vi "EdgeDetection-Simple.vi"() -> ()   [LabVIEW 2014]
doc: "This example shows how to use the Edge Tool in NI Vision. The Edge Tool finds edges (or sharp transitions in the pixels values) along a given line or ROI profile. The Edge Tool is a precursor function to many of the gauging and inspection tasks. For example, the location of the edges found along a line profile across an object can interpreted as the boundaries of the object whose dimensions have to be measured for a gauging application or the presence of a crack in the surface of an object for an inspection application."
uses:
  <vilib>/vision/NI_Vision_Development_Module.lvlib
panel:
  in  "Process":u16(ring)=2 items=["Get First Edge", "Get First + Last Edge", "Get All Edges"]
  in  "Threshold Parameters":T1={"Level Type"=enum."Absolute Value", "Threshold Level"=200, "Hysteresis"=10}
  out "Number of Edges Detected":i32
  out "Image":T2(plugin-control)
  out "Line Profile":cluster{"x0":sgl, "dx":sgl, "Pixels Line":sgl[]}(graph)
  in  "Stop":bool
  # "Instruction:\nThreshold Level can be either absolute or relative. \nAbsolute threshold is based on the pixel values. \nRelative threshold is expressed as a percentage of the pixel-value range found along the path defined by the pixel coordinates."
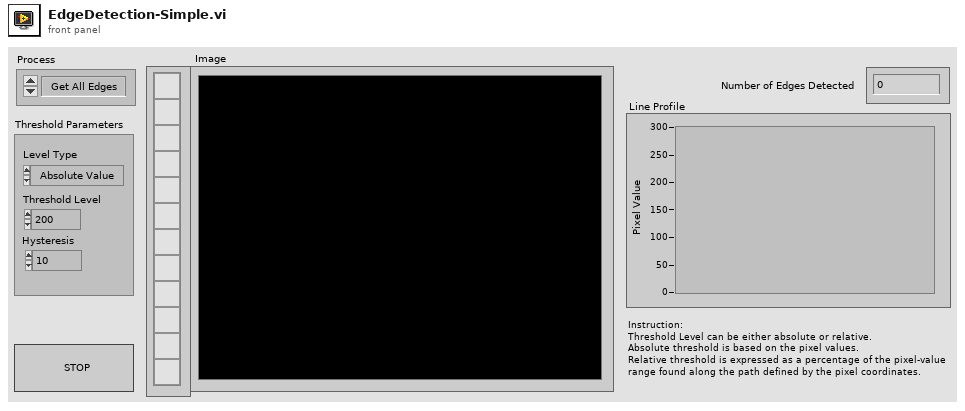
[diagram p1: front panel]
types:
  T1 = cluster{"Level Type":enum32{"Absolute Value", "Relative value"}, "Threshold Level":i32, "Hysteresis":i32}
  T2 = typedef "IMAQ Image.ctl" = refnum<image>
  T3 = typedef "IMAQ Line" = cluster{"Start X":i32, "Start Y":i32, "End X":i32, "End Y":i32}
  T4 = typedef "ROI Descriptor" = cluster{"Global Rectangle":i32[], "Contours":cluster{"ID":enum32{"External", "Internal"}, "Type":u32, "Coordinates":i32[]}[]}
  T5 = cluster{"Global Rectangle":i32[], "Contours":cluster{"Contour Type":u32, "ROI Type":u32, "Points":i32[]}[]}
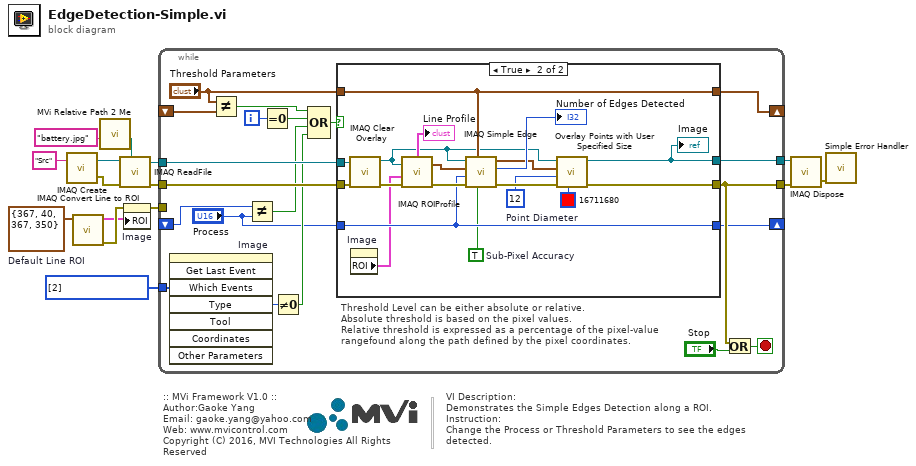
[diagram p0: block diagram]
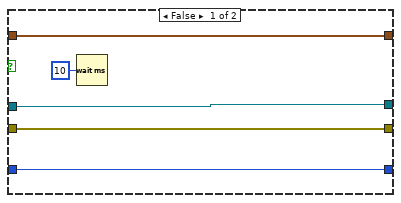
[diagram p2: hidden frame]
diagram:
  w4 = i32[] [2] items=["No Event"=0, "Click Event"=1, "Draw Event"=2, "Size Event"=4, "Scroll Event"=5, "Double Click Event"=8] ("Which Events")
  w7 = T3 {"Start X"=367, "Start Y"=40, "End X"=367, "End Y"=350}  # Default Line ROI
  # "VI Description:\nDemonstrates the Simple Edges Detection along a ROI.\nInstruction:\nChange the Process or Threshold Parameters to see the edges detected."
  # ":: MVi Framework V1.0 ::\nAuthor:Gaoke Yang\nEmail: gaoke.yang@yahoo.com\nWeb: www.mvicontrol.com\nCopyright (C) 2016, MVI Technologies All Rights Reserved"
  n1 = call "IMAQ Create"("Image Name"="Src") -> ("New Image"=w14:T2, "error out"=w13:errorcluster)  [unwired: 4 in]
  n2 = call "IMAQ Convert Line to ROI"("Line"=w7) -> ("error out"=w3:errorcluster, "ROI Descriptor"=w2:T4)  [unwired: 8 in]
  n3 = call "MVi Relative Path 2 Me.vi"("Relative Path"="battery.jpg" ("name or relative path")) -> ("Appended Dir"=w5:path)  [unwired: 5 in, 1 out]
  n4 = call "IMAQ ReadFile"("File Path"=w5, "error in (no error)"=w13, "Image"=w14) -> ("error out"=w8:errorcluster, "Image Out"=w9:T2)  [unwired: 4 in, 3 out]
  n5 = property on="Image" class="ImageControl"(error in=w3, "ROI"=w2) -> (error out=w1:errorcluster)  [unwired: 1 in, 1 out]
  n6 = while {
    tunnel: w9 -> [w34]
    tunnel: w8 -> [w35]
    tunnel: [w30] -> w12
    tunnel: [w31] -> w11
    shift-right: [w28] -> _
    shift-left: _ -> [w26]
    shift-right: [w25] -> _
    shift-left: _ -> [w19]
    tunnel: w4 -> [w24]
    tunnel: w1 -> [_]
    i -> [w29]
    stop <- w32 stop-if-true
    # "Threshold Level can be either absolute or relative. \nAbsolute threshold is based on the pixel values. \nRelative threshold is expressed as a percentage of the pixel-value\nrangefound along the path defined by the pixel coordinates."
    n7 = invoke on="Image" class="ImageControl" method="Get Last Event"("Which Events"=w24) -> ("Type"=w23:i32)  [unwired: 7 in, 7 out]
    n8 = Not Equal?(x="Threshold Parameters", y=w26) -> (x != y?=w20:bool)
    n9 = Not Equal?(x=w19, y="Process") -> (x != y?=w16:bool)
    n10 = Equal To 0?(x=w29) -> (x = 0?=w17:bool)
    n11 = Not Equal To 0?(x=w23) -> (x != 0?=w21:bool)
    n12 = Compound Arithmetic op=OR(w20, w17, w16, w21) -> (w22:bool)
    n13 = case shown="True" w22 {
      tunnel: w35 -> [w39 w47]
      tunnel: w34 -> [w40 w48]
      tunnel: [w40 w49] -> w31
      tunnel: [w39 w51] -> w30
      tunnel: "Threshold Parameters" -> [w37 w56]
      tunnel: [w37 w56] -> w28
      tunnel: "Process" -> [w36 w43]
      tunnel: [w36 w43] -> w25
      frame False {
        n14 = Wait (ms)(milliseconds to wait=u32 10) -> ()  [unwired: 1 out]
      }
      frame True {
        w42 = TRUE  # Sub-Pixel Accuracy
        w44 = u32 12  # Point Diameter
        n15 = call "IMAQ Clear Overlay"("error in (no error)"=w47, "Image"=w48) -> ("error out"=w46:errorcluster, "Image Out"=w45:T2)  [unwired: 8 in]
        n16 = property on="Image" class="ImageControl"() -> ("ROI"=w41:T5)  [unwired: 2 in, 2 out]
        n17 = call "IMAQ ROIProfile"("error in (no error)"=w46, "ROI Descriptor"=w41, "Image"=w45) -> ("error out"=w57:errorcluster, "ROI Graph"=→"Line Profile":cluster{"x0":sgl, "dx":sgl, "Pixels Line":sgl[]}, "Pixel Coordinates"=w55:cluster{"X":u32, "Y":u32}[])  [unwired: 1 in, 2 out]
        n18 = call "IMAQ Simple Edge"("Sub-Pixel Accuracy"=w42, "Threshold Parameters"=w56, "error in (no error)"=w57, "Process"=w43, "Pixel Coordinates"=w55, "Image Src"=w45) -> ("error out"=w50:errorcluster, "Number of Edges"=→"Number of Edges Detected":i32, "Edges Coordinates"=w52:cluster{"X":sgl, "Y":sgl}[])  [unwired: 3 in]
        n19 = call "Overlay Points with User Specified Size.vi"("Color"=u32 16711680, "error in"=w50, "Point Diameter (5)"=w44, "Points"=w52, "Image In"=w45) -> ("error out"=w51:errorcluster, "Image Out"=w49:T2)  [unwired: 5 in]
        "Image" <- w49
      }
    }
    n20 = Or(x=w30, y="Stop") -> (x .or. y?=w32:bool)
  }
  n21 = call "IMAQ Dispose"("Image"=w11, "error in (no error)"=w12) -> ("error out"=w10:errorcluster)  [unwired: 4 in]
  n22 = call <vilib>:"Simple Error Handler.vi"("error in (no error)"=w10) -> ()  [unwired: 4 in, 5 out]
